vi "Attach Metadata to TDMS.vi"(8 "error in (no error)":errorcluster, 11 "experiment folder":path) -> (0 "error out":errorcluster, 2 "file path out":path)   [LabVIEW 2016]
uses:
  <userlib>/_OpenG.lib/file/file.llb/Build Path - Traditional__ogtk.vi
  <userlib>/LevyLab/LV to ITX/Data/Data.lvclass
panel:
  out "group/channel names":string[][](array[string])
  out "group names":string[](array[string])
  out "device details":string[][](array[string])
  out "wiring":string[][](array[string])
  out "Experiment Parameters From 1st ITX":T1
  out "data":T2
  out "Notes":string
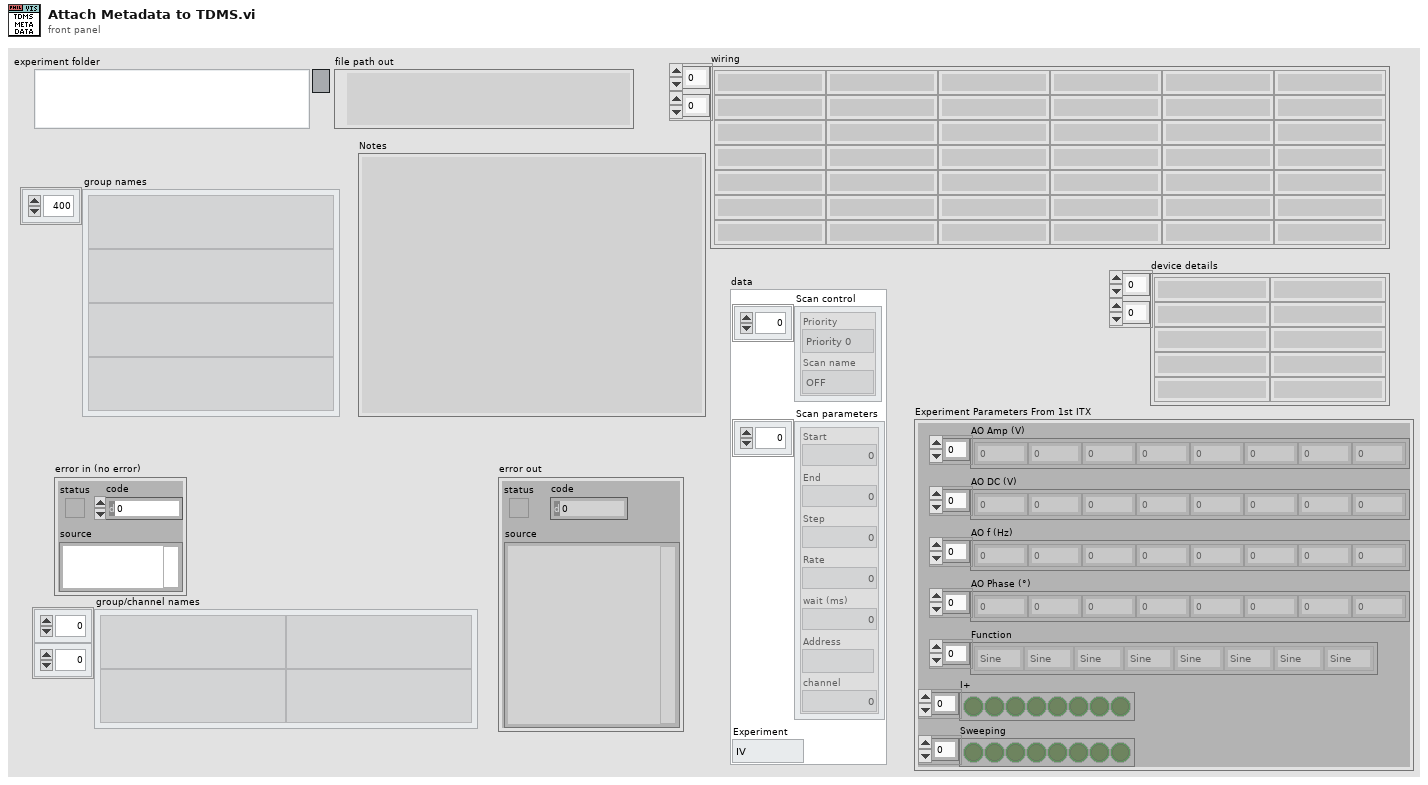
[diagram p1: front panel]
types:
  T1 = cluster{"AO Amp (V)":dbl[], "AO DC (V)":dbl[], "AO f (Hz)":dbl[], "AO Phase (°)":dbl[], "Function":enum16{"Sine", "Triangle", "Square", "Sawtooth"}[], "I+":bool[], "Sweeping":bool[]}
  T2 = cluster{"Scan control":cluster{"Priority":enum16{"Priority 0", "Priority 1", "Priority 2", "Priority 3", "Priority 4", "Priority 5"}, "Scan name":enum16{"OFF", "DSA_Vsg2", "DSA_Vsg3", "DSA_Vbg", "DSA_Vsg1", "DSA_freq", "DSA_Vamp", "time", "Lockin Amplitude", "Lockin Frequency", "Lockin Bias", "Delay", "Strain", "DAQ Bias", "Magnet Field", "Temperature", "MW f1", "MW f2", "MW Amplitude1", "MW Amplitude2"}}[], "Scan parameters":cluster{"Start":dbl, "End":dbl, "Step":dbl, "Rate":dbl, "wait (ms)":u32, "Address":string, "channel":i32}[], "Experiment":enum16{"IV", "IV_Fast", "IV_Sweep", "THz_DelayLine", "Lockin_Vsg", "Lockin_Sweep", "Lockin_Time", "AI WFM time", "Lockin (experimental)"}}
  T3 = enum16{"open", "open or create", "create or replace", "create", "open (read-only)"}
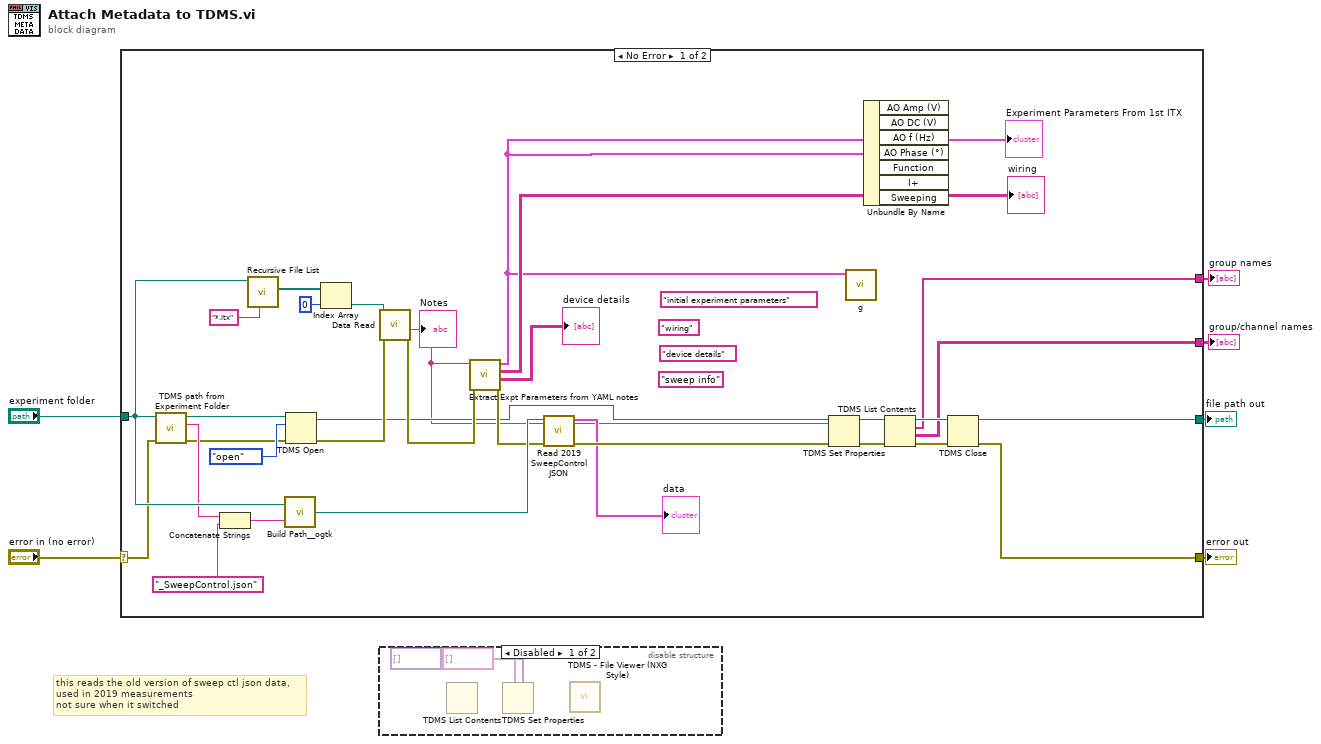
[diagram p0: block diagram]
diagram:
  # "this reads the old version of sweep ctl json data,\nused in 2019 measurements\nnot sure when it switched"
  n1 = case shown="No Error" "error in (no error)" {
    selector: "error in (no error)" -> [w9 w38]
    tunnel: [w36 w38] -> w5
    tunnel: [w35 _] -> w4
    tunnel: "experiment folder" -> [w27 _]
    tunnel: [w11 _] -> w2
    tunnel: [w10 _] -> w1
    frame No Error {
      (unwired) "sweep info"
      (unwired) "device details"
      (unwired) "wiring"
      (unwired) "initial experiment parameters"
      n2 = call "TDMS path from Experiment Folder.vi"("error in (no error)"=w9, "experiment folder"=w27) -> ("error out"=w8:errorcluster, "name"=w25:string, "tdms file path"=w30:path)  [unwired: 7 in]
      n3 = Concatenate Strings(w25, "_SweepControl.json" ("string")) -> (w26:string)
      n4 = call <vilib>:"Recursive File List.vi"("pattern"="*.itx", "Folder Path"=w27) -> ("All Files in Dir"=w34:path[])  [unwired: 5 in, 4 out]
      n5 = call-poly <userlib>:"Build Path__ogtk.vi"("name or relative path"=w26, "base path"=w27) -> ("appended path"=w23:path)
      n6 = TDMS Open(8:w8, 10:T3."open" ("operation (0:open)"), 11:w30) -> (0:w31:errorcluster, 3:w19:refnum<k34>)  [unwired: 4 in]
      n7 = Index Array(array=w34, index=0) -> (element=w32:path)
      n8 = call <userlib>:"Data Read.vi"("error in (no error)"=w31, "path"=w32) -> ("error out"=w28:errorcluster, "Notes"=w7:string)  [unwired: 6 in, 2 out]
      "Notes" <- w7
      n9 = call "Extract Expt Parameters from YAML notes.vi"("error in (no error)"=w28, "YAML Comments IN"=w7) -> ("error out"=w22:errorcluster, "device details"=→"device details":string[][], "wiring"=→"wiring":string[][], "Experiment Parameters From 1st ITX"=w16:T1)  [unwired: 6 in]
      "Experiment Parameters From 1st ITX" <- w16
      n10 = call "Read 2019 SweepControl JSON.vi"("error in (no error)"=w22, "json file"=w23) -> ("error out"=w18:errorcluster, "data"=→"data":T2)  [unwired: 8 in]
      n11 = TDMS Set Properties(5:w7, 7:w7, 8:w18, 11:w19) -> (0:w14:errorcluster, 3:w13:refnum<k34>)  [unwired: 2 in, 2 out]
      n12 = call "g.vi"("Experiment Parameters From 1st ITX"=w16) -> ()  [unwired: 11 in]
      n13 = Unbundle By Name(w16) -> ()  [unwired: 7 out]
      n14 = TDMS List Contents(4:w14, 7:w13) -> (0:w15:errorcluster, 1:w11:string[][], 2:w10:string[], 3:w17:refnum<k34>)  [unwired: 1 in]
      n15 = TDMS Close(8:w15, 11:w17) -> (0:w36:errorcluster, 3:w35:path)
    }
    frame Error {
    }
  }
  "error out" <- w5
  "file path out" <- w4
  "group/channel names" <- w2
  "group names" <- w1
  n16 = disable-structure shown="Disabled" {
    frame Disabled {
      n17 = TDMS List Contents() -> ()  [unwired: 3 in, 4 out]
      n18 = TDMS Set Properties(5:variant[] [] ("property values"), 7:string[] [] ("property names")) -> ()  [unwired: 4 in, 4 out]
      n19 = call <vilib>:"TDMS - File Viewer (NXG Style).vi"() -> ()  [unwired: 10 in, 2 out]
    }
    frame Enabled {
    }
  }
